vi "TildaPassiveAcqOneStep.vi"(9 "nOfBins":u32) -> (0 "abortOrTimeOut":bool)   [LabVIEW 2014]
uses:
  <vilib>/Platform/TimedLoop/XDataNode/timing_clust.ctl
  <vilib>/Platform/TimedLoop/XDataNode/nitl_modes.ctl
  <vilib>/Platform/TimedLoop/XDataNode/wakeup.ctl
  Controls/triggerEdge.ctl
  Controls/infoHandle.ctl
  <vilib>/rvi/Emulation/niFpgaSctlEmulationGetInTimedLoop.vi
  <vilib>/rvi/Emulation/niFpgaEmulationReportErrorSimple.vi
  <vilib>/rvi/Emulation/niFpgaGetClockAttributes.vi
  <vilib>/rvi/Emulation/niFpgaCriticalErrorInLSC.vi
  Sequencer/sequencerGlobVars.vi
  <vilib>/rvi/eio/common/nirviEmuTemplateMethod_errors.vi
  <vilib>/Platform/TimedLoop/XDataNode/XDataNode.xnode
  <vilib>/eio/EIONode/EIONode.xnode
  <vilib>/Platform/TimedLoop/XDataNode/XDNodeRunTimeDep.lvlib
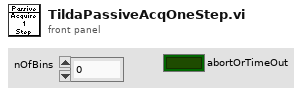
[diagram p1: front panel]
types:
  T1 = typedef "XDNodeRunTimeDep.lvlib/timing_clust.ctl" = cluster{"Expected End [f-1]":u64, "Actual End [f-1]":u64, "Finished Late? [f-1]":bool, "Expected End [i-1]":u64, "Actual End [i-1]":u64, "Finished Late? [i-1]":bool, "Expected Start [i]":u64, "Actual Start [i]":u64, "Expected Start [f]":u64, "Actual Start [f]":u64, "Source Name":string, "Structure Name":string, "Period":i64, "Deadline":i64, "Offset":i64, "Start":i64, "Priority":i32, "Timeout":i32, "Mode":T2, "Wakeup Reason":T3, "Error":errorcluster, "Source Type":string, "Secondary Source Type":string, "Global End Time":u64, "Global Start Time":u64, "Frame Duration":u64, "Iteration Duration":u64, "Assigned CPU":i32, "I/O Scan Engine Mode":u32}
  T2 = typedef "XDNodeRunTimeDep.lvlib/nitl_modes.ctl" = enum32{"No Change", "Process missed periods, maintain original phase", "Discard missed periods, maintain original phase", "Process missed periods, ignore original phase", "Discard missed periods, ignore original phase"}
  T3 = typedef "XDNodeRunTimeDep.lvlib/wakeup.ctl" = enum32{"Normal", "Aborted", "Asynchronous wakeup", "Timing source error", "Timed loop error", "Timeout"}
  T4 = typedef "triggerEdge.ctl" = enum8{"either", "false-true", "true-false"}
  T5 = typedef "infoHandle.ctl" = enum16{"abortedScan", "stepComplete", "newScan", "newBunch"}
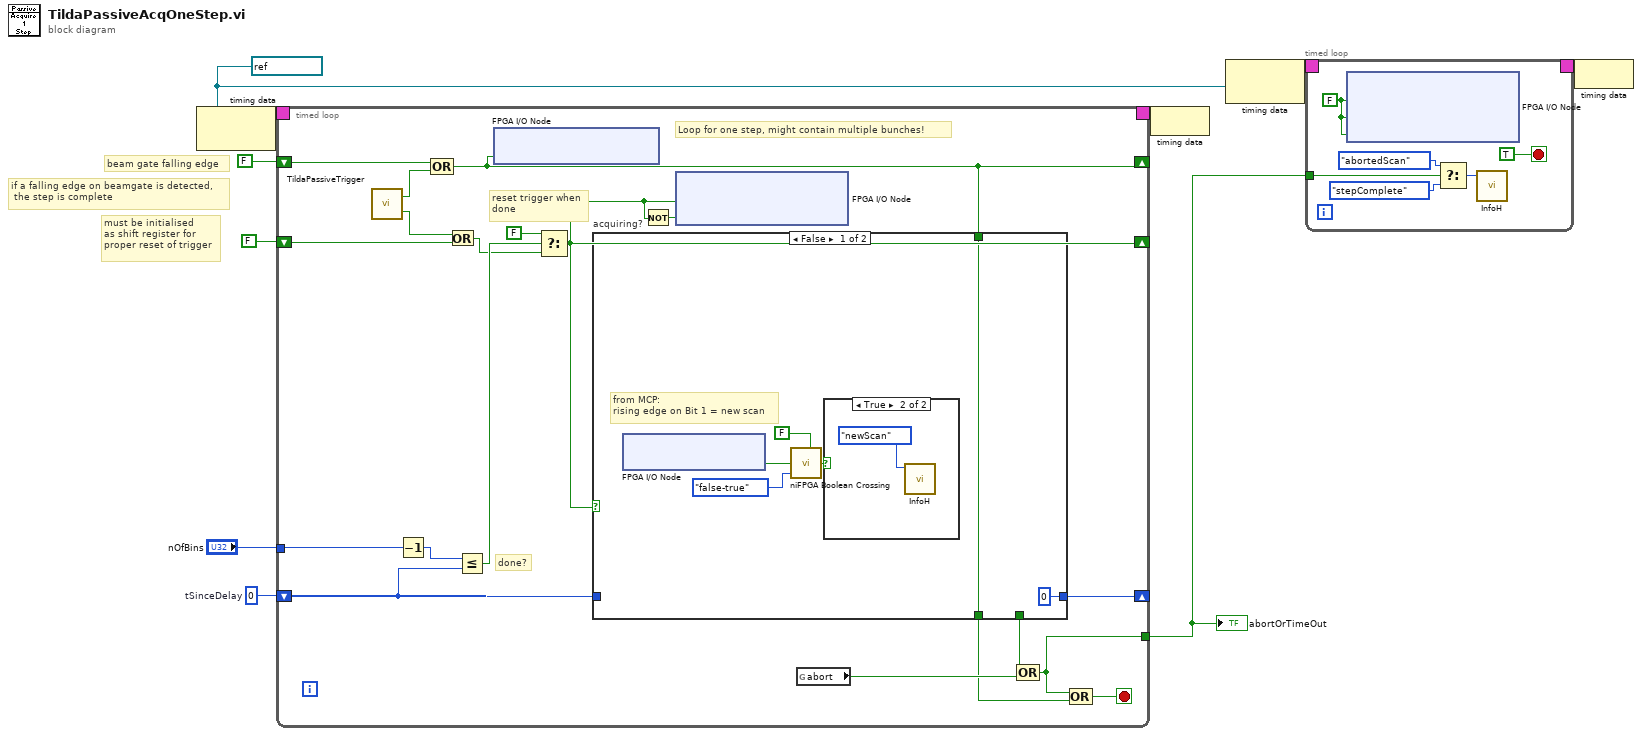
[diagram p0: block diagram]
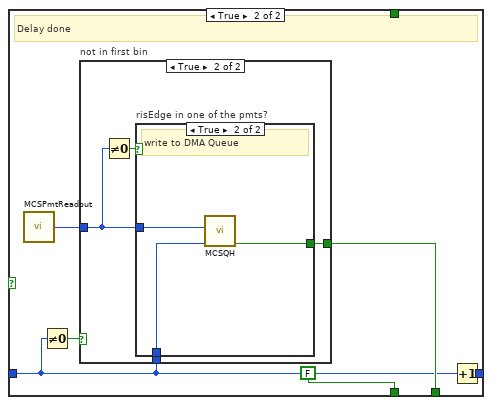
[diagram p3: hidden frame]
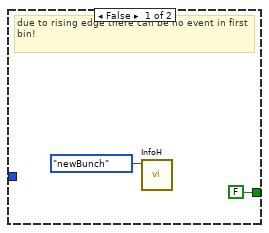
[diagram p4: hidden frame]
diagram:
  w6 = u32 0  # tSinceDelay
  w4 = refnum<k21> "100MHz" ("Source Name")
  # "if a falling edge on beamgate is detected,\n the step is complete"
  # "beam gate falling edge"
  # "must be initialised\nas shift register for\nproper reset of trigger"
  n1 = node-c288(w4) -> (w10:T1)
  n2 = timed-loop {
    timing: w10 -> [_]
    timing-out: [_] -> w9
    shift-right: [w29] -> _
    shift-left: w6 -> [w26]
    tunnel: "nOfBins" -> [w28]
    tunnel: [w22] -> w3
    shift-right: [w11] -> _
    shift-left: FALSE ("triggered") -> [w21]
    shift-right: [w13] -> _
    shift-left: FALSE ("crossing") -> [w16]
    stop <- w23 stop-if-true
    # "reset trigger when\ndone"
    # "Loop for one step, might contain multiple bunches!"
    # "done?"
    n3 = call "TildaPassiveTrigger.vi"() -> ("beamGateFallingEdge"=w15:bool, "triggered"=w14:bool)  [unwired: 18 in]
    n4 = Decrement(x=w28) -> (x-1=w27:u32)
    n5 = Compound Arithmetic op=OR(w16, w15) -> (w13:bool)
    n6 = Or(x=w14, y=w21) -> (x .or. y?=w19:bool)
    n7 = Less Or Equal?(x=w27, y=w26) -> (x <= y?=w20:bool)
    n8 = xnode "FPGA I/O Node"("bg8FallEdgeDio12Con1"=w13) -> ()  [unwired: 1 in, 1 out]
    n9 = Select(t=FALSE, s=w20, f=w19) -> (s? t:f=w11:bool)
    n10 = case "acquiring?" shown="False" w11 {
      tunnel: w26 -> [_ w37]
      tunnel: [u32 0 w42] -> w29
      tunnel: [_ w40] -> w25
      tunnel: [w34 FALSE ("Connector1/DIO25")] -> w17
      tunnel: w13 -> [w34 _]
      frame False {
        # "from MCP:\nrising edge on Bit 1 = new scan"
        n11 = xnode "FPGA I/O Node"() -> ("Connector1/DIO26"=w32:bool)  [unwired: 1 in, 1 out]
        n12 = call <vilib>:"niFPGA Boolean Crossing.vi"("input"=w32, "triggerEdge"=triggerEdge."false-true", "initialize"=FALSE) -> ("crossing"=w33:bool)  [unwired: 6 in]
        n13 = case shown="True" w33 {
          frame False {
          }
          frame True {
            n14 = call "InfoH.vi"("info"=infoHandle."newScan") -> ()  [unwired: 11 in]
          }
        }
      }
      frame True {
        # "Delay done"
        n15 = call "MCSPmtReadout.vi"() -> ("pmtOut"=w41:u8)  [unwired: 5 in]
        n16 = Not Equal To 0?(x=w37) -> (x != 0?=w38:bool)
        n17 = case "not in first bin" shown="True" w38 {
          tunnel: w41 -> [_ w47]
          tunnel: w37 -> [_ w46]
          tunnel: [FALSE ("MCSWriteTimeout") w45] -> w40
          frame False {
            # "due to rising edge there can be no event in first bin!"
            n18 = call "InfoH.vi"("info"=infoHandle."newBunch") -> ()  [unwired: 11 in]
          }
          frame True {
            n19 = Not Equal To 0?(x=w47) -> (x != 0?=w48:bool)
            n20 = case "risEdge in one of the pmts?" shown="True" w48 {
              tunnel: w47 -> [_ w50]
              tunnel: w46 -> [_ w51]
              tunnel: [_ w49] -> w45
              frame False {
              }
              frame True {
                # "write to DMA Queue"
                n21 = call "MCSQH.vi"("TimeStamp"=w51, "activePMT"=w50) -> ("MCSWriteTimeout"=w49:bool)  [unwired: 9 in]
              }
            }
          }
        }
        n22 = Increment(x=w37) -> (x+1=w42:u32)
      }
    }
    n23 = Not(x=w11) -> (.not. x?=w12:bool)
    n24 = xnode "FPGA I/O Node"("MCSScanFlagDio9Con1"=w11, "triggerArmedDio13Con1"=w12) -> ()  [unwired: 2 in, 2 out]
    n25 = global read "sequencerGlobVars.vi" "abort"() -> (w24:bool)
    n26 = Compound Arithmetic op=OR(w25, w24) -> (w22:bool)
    n27 = Compound Arithmetic op=OR(w22, w17) -> (w23:bool)
  }
  "abortOrTimeOut" <- w3
  n28 = node-c288(w9) -> ()
  n29 = node-c288(w4) -> (w8:T1)
  n30 = timed-loop {
    timing: w8 -> [_]
    timing-out: [_] -> w7
    tunnel: w3 -> [w58]
    stop <- TRUE stop-if-true
    w54 = FALSE ("MCSScanFlagDio9Con1")
    n31 = xnode "FPGA I/O Node"("MCSScanFlagDio9Con1"=w54, "bg8FallEdgeDio12Con1"=w54, "triggerArmedDio13Con1"=w54) -> ()  [unwired: 3 in, 3 out]
    n32 = Select(t=infoHandle."abortedScan" ("info"), s=w58, f=infoHandle."stepComplete" ("info")) -> (s? t:f=w55:T5)
    n33 = call "InfoH.vi"("info"=w55) -> ()  [unwired: 11 in]
  }
  n34 = node-c288(w7) -> ()
